vi "FPGA_CounterReadOutput.vi"(8 "error in (no error)":errorcluster, 11 "Ctr Ref in":T1) -> (0 "error out":errorcluster, 1 "Direction":bool, 2 "Value":i32, 3 "Ctr Ref out":T1)   [LabVIEW 2017]
uses:
  <vilib>/Rock Robotics/SystemInterfaces/Counter/FPGA_CounterCtrDevRef.ctl
  <vilib>/Rock Robotics/SystemInterfaces/Counter/FPGA_CounterCtrSystemIndex.ctl
  <vilib>/Rock Robotics/SystemInterfaces/System/FPGA_SystemFPGA Ref Global.vi
  <vilib>/Utility/error.llb/Error Cluster From Error Code.vi
  <vilib>/rvi/errors/niLvFpgaAdjustHostInterfaceError.vi
  <vilib>/rvi/interface/nirviReadWriteControl/nirviReadWriteControl.xnode
  <vilib>/Rock Robotics/SystemInterfaces/System/FPGA_SystemFRC FPGA Ref.ctl
  NiFpgaLv.dll
  <vilib>/rvi/interface/Simulation/niFpgaSimulationCallBeginRW.vi
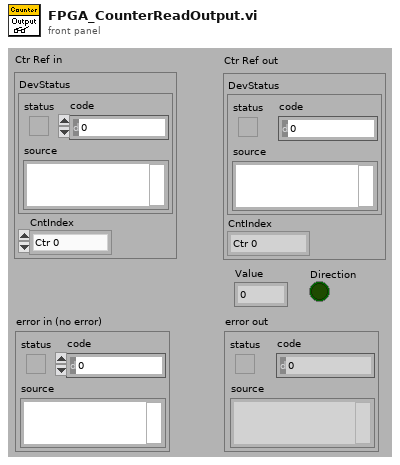
[diagram p1: front panel]
types:
  T1 = typedef "FPGA_CounterCtrDevRef.ctl" = cluster{"DevStatus":errorcluster, "CntIndex":T2}
  T2 = typedef "FPGA_CounterCtrSystemIndex.ctl" = enum8{"Ctr 0", "Ctr 1", "Ctr 2", "Ctr 3", "Ctr 4", "Ctr 5", "Ctr 6", "Ctr 7", "Invalid"}
  T3 = typedef "FPGA_SystemFRC FPGA Ref.ctl" = refnum<k20>
  T4 = cluster{"Direction":bool, "Value":fxp<+/-,31,31>}
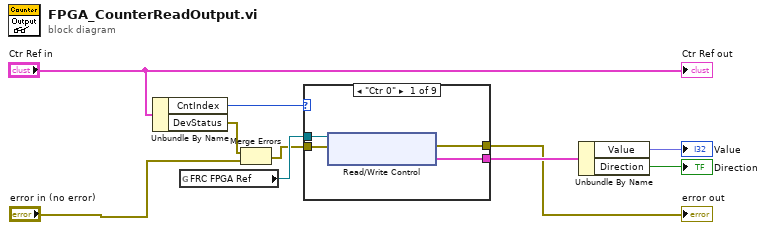
[diagram p0: block diagram]
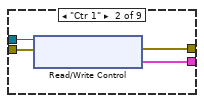
[diagram p2: hidden frame]
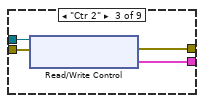
[diagram p3: hidden frame]
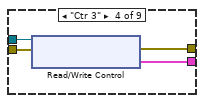
[diagram p4: hidden frame]
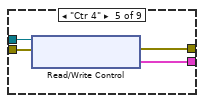
[diagram p5: hidden frame]
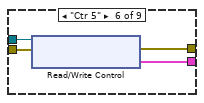
[diagram p6: hidden frame]
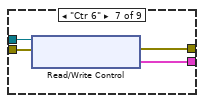
[diagram p7: hidden frame]
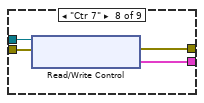
[diagram p8: hidden frame]
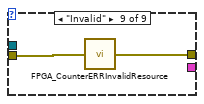
[diagram p9: hidden frame]
diagram:
  n1 = Unbundle By Name("Ctr Ref in") -> ("CntIndex"=w5:T2, "DevStatus"=w3:errorcluster)
  n2 = global read "FPGA_SystemFPGA Ref Global.vi" "FRC FPGA Ref"() -> (w4:T3)
  n3 = Merge Errors(w3, "error in (no error)") -> (w2:errorcluster)
  n4 = case shown="\"Ctr 0\"" w5 {
    tunnel: w4 -> [w13 w18 w22 w26 w30 w34 w38 w42 _]
    tunnel: w2 -> [w14 w17 w21 w25 w29 w33 w37 w41 w43]
    tunnel: [w12 w16 w20 w24 w28 w32 w36 w40 w44] -> w8
    tunnel: [w11 w15 w19 w23 w27 w31 w35 w39 _] -> w10
    frame "Ctr 0" {
      n5 = xnode "Read/Write Control"("FPGA VI Reference In"=w13, "error in"=w14) -> ("error out"=w12:errorcluster, "Counter0.Output"=w11:T4)  [unwired: 1 out]
    }
    frame "Ctr 1" {
      n6 = xnode "Read/Write Control"("FPGA VI Reference In"=w18, "error in"=w17) -> ("error out"=w16:errorcluster, "Counter1.Output"=w15:T4)  [unwired: 1 out]
    }
    frame "Ctr 2" {
      n7 = xnode "Read/Write Control"("FPGA VI Reference In"=w22, "error in"=w21) -> ("error out"=w20:errorcluster, "Counter2.Output"=w19:T4)  [unwired: 1 out]
    }
    frame "Ctr 3" {
      n8 = xnode "Read/Write Control"("FPGA VI Reference In"=w26, "error in"=w25) -> ("error out"=w24:errorcluster, "Counter3.Output"=w23:T4)  [unwired: 1 out]
    }
    frame "Ctr 4" {
      n9 = xnode "Read/Write Control"("FPGA VI Reference In"=w30, "error in"=w29) -> ("error out"=w28:errorcluster, "Counter4.Output"=w27:T4)  [unwired: 1 out]
    }
    frame "Ctr 5" {
      n10 = xnode "Read/Write Control"("FPGA VI Reference In"=w34, "error in"=w33) -> ("error out"=w32:errorcluster, "Counter5.Output"=w31:T4)  [unwired: 1 out]
    }
    frame "Ctr 6" {
      n11 = xnode "Read/Write Control"("FPGA VI Reference In"=w38, "error in"=w37) -> ("error out"=w36:errorcluster, "Counter6.Output"=w35:T4)  [unwired: 1 out]
    }
    frame "Ctr 7" {
      n12 = xnode "Read/Write Control"("FPGA VI Reference In"=w42, "error in"=w41) -> ("error out"=w40:errorcluster, "Counter7.Output"=w39:T4)  [unwired: 1 out]
    }
    frame "Invalid" {
      n13 = call <vilib>:"FPGA_CounterERRInvalidResource.vi"("error in (no error)"=w43) -> ("error out"=w44:errorcluster)
    }
  }
  "error out" <- w8
  n14 = Unbundle By Name(w10) -> ("Value"=→"Value":fxp<+/-,31,31>, "Direction"=→"Direction":bool)
  "Ctr Ref out" <- "Ctr Ref in"
